vi "Write Payload.vi"(10 "Payload":string, 11 "GDSII.DataType.Real in":refnum<class "GDSII.DataType.Real.lvclass">) -> (3 "GDSII.DataType.Real out":refnum<class "GDSII.DataType.Real.lvclass">)   [LabVIEW 2019, in "GDSII.DataType.Real.lvclass"]
uses:
  GDSII.DataType.Real.lvclass
  GDSII.DataType.Real.lvclass/GDSII.DataType.Real.ctl
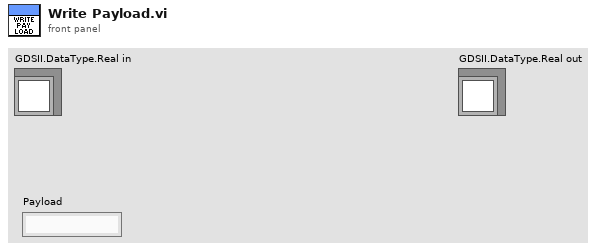
[diagram p1: front panel]
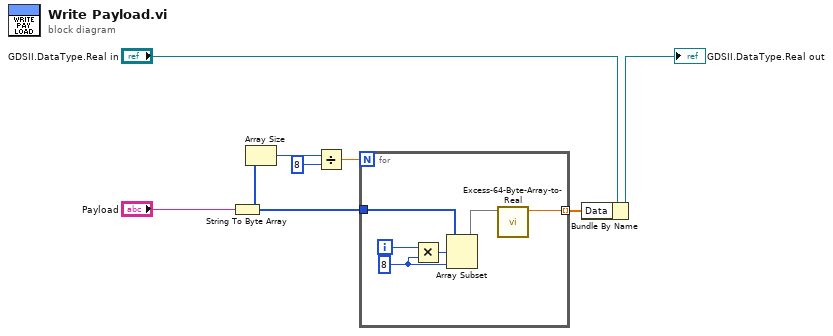
[diagram p0: block diagram]
diagram:
  n1 = String To Byte Array(string="Payload") -> (unsigned byte array=w5:u8[])
  n2 = Array Size(array=w5) -> (size(s)=w8:i32)
  n3 = Divide(x=w8, y=8) -> (x/y=w6:dbl)
  n4 = for {
    N: w6 -> [_]
    tunnel: w5 -> [w10]
    tunnel: [w9] -> w1 mode=indexing
    i -> [w14]
    w11 = 8 ("y")
    n5 = Multiply(x=w14, y=w11) -> (x*y=w12:i32)
    n6 = Array Subset(array=w10, index=w12, length=w11) -> (w13:u8[])
    n7 = call "Excess-64-Byte-Array-to-Real.vi"("Byte array (4 or 8 bytes)"=w13) -> ("Real Number"=w9:dbl)  [unwired: 10 in]
  }
  n8 = Bundle By Name(cluster="GDSII.DataType.Real in", "Data"=w1) -> (→"GDSII.DataType.Real out":refnum<class "GDSII.DataType.Real.lvclass">)
